vi "provide_OME_manufacturer_spec.vi"(4 "id chain":string[](array[string]), 6 "key chain":string[](array[string]), 8 "error in (no error)":errorcluster, 10 "XMLElement in":refnum<class "XMLElement.lvclass">, 11 "GenericPlugin in":refnum<class "GenericComponent.lvclass">) -> (0 "error out":errorcluster, 2 "XMLElement out":refnum<class "XMLElement.lvclass">, 3 "GenericPlugin out":refnum<class "GenericComponent.lvclass">)   [LabVIEW 2010, in "GenericComponent.lvclass"]
uses:
  GenericComponent.lvclass
  XMLElement/XMLElement/XMLElement.lvclass
  GenericComponent.lvclass/GenericComponent.ctl
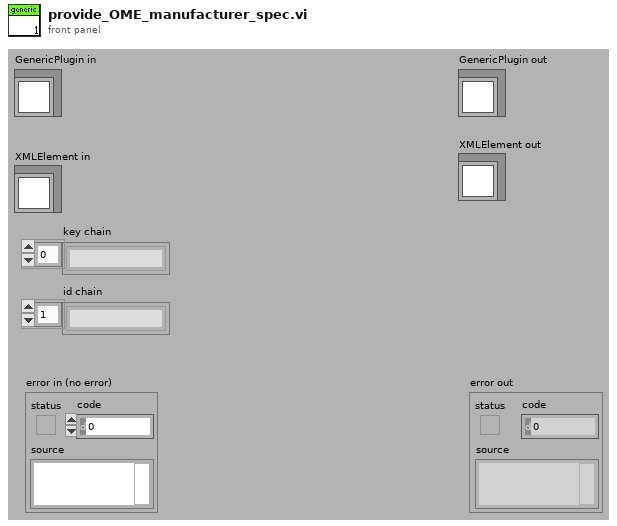
[diagram p1: front panel]
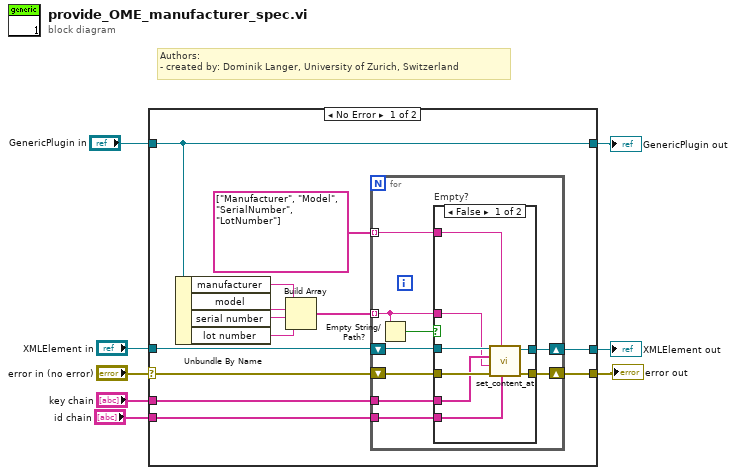
[diagram p0: block diagram]
diagram:
  # "Authors: \n- created by: Dominik Langer, University of Zurich, Switzerland"
  n1 = case shown="No Error" "error in (no error)" {
    selector: "error in (no error)" -> [w20 w43]
    tunnel: [w19 w43] -> w7
    tunnel: [w9 w42] -> w5
    tunnel: "GenericPlugin in" -> [w9 w42]
    tunnel: "XMLElement in" -> [w21 w41]
    tunnel: "key chain" -> [w12 _]
    tunnel: "id chain" -> [w11 _]
    tunnel: [w10 w41] -> w1
    frame No Error {
      n2 = Unbundle By Name(w9) -> ("manufacturer"=w17:string, "model"=w16:string, "serial number"=w15:string, "lot number"=w18:string)
      n3 = Build Array(w17, w16, w15, w18) -> (w14:string[])
      n4 = for {
        tunnel: w14 -> [w27] mode=indexing
        shift-right: [w28] -> w19
        shift-left: w20 -> [w29]
        tunnel: string[] ["Manufacturer", "Model", "SerialNumber", "LotNumber"] -> [w25] mode=indexing
        tunnel: w12 -> [w24]
        tunnel: w11 -> [w23]
        shift-right: [w22] -> w10
        shift-left: w21 -> [w30]
        n5 = Empty String/Path?(string/path=w27) -> (empty?=w26:bool)
        n6 = case "Empty?" shown="False" w26 {
          tunnel: w30 -> [w38 w39]
          tunnel: w29 -> [w37 w40]
          tunnel: [w36 w40] -> w28
          tunnel: w27 -> [w32 _]
          tunnel: w25 -> [w31 _]
          tunnel: w24 -> [w35 _]
          tunnel: w23 -> [w33 _]
          tunnel: [w34 w39] -> w22
          frame False {
            n7 = call "set_content_at.vi"("id chain"=w33, "attribute name"=w31, "error in (no error)"=w37, "content"=w32, "key chain"=w35, "Element in"=w38) -> ("error out"=w36:errorcluster, "Element out"=w34:refnum<class "XMLElement.lvclass">)  [unwired: 4 in]
          }
          frame True {
          }
        }
      }
    }
    frame Error {
    }
  }
  "error out" <- w7
  "GenericPlugin out" <- w5
  "XMLElement out" <- w1
